vi "S2C_InitMenuItems.vi"(8 "Error In":errorcluster) -> (0 "Error Out":errorcluster)   [LabVIEW 2015]
doc: "Toggles the \"Local File\" runtime menu item."
uses:
  Globals/S2C_Globals.vi
  Globals/S2C_GlobalMenus.vi
  LVIS/Sub VIs/Globals/LVIS_DcGlobals.vi
  XML/S2C_XML_Globals.vi
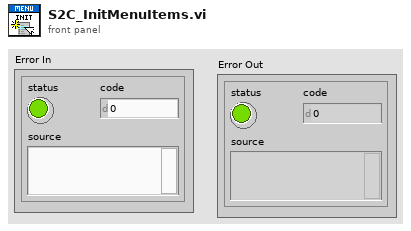
[diagram p1: front panel]
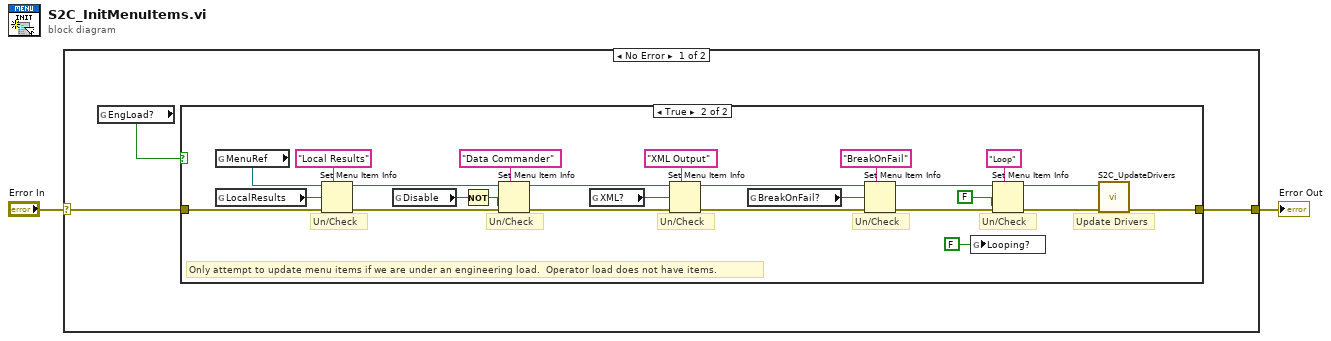
[diagram p0: block diagram]
diagram:
  n1 = case shown="No Error" "Error In" {
    selector: "Error In" -> [w5 w32]
    tunnel: [w4 w32] -> w1
    frame No Error {
      n2 = global read "S2C_Globals.vi" "EngLoad?"() -> (w3:bool)
      n3 = case shown="True" w3 {
        tunnel: w5 -> [w6 w24]
        tunnel: [w6 w23] -> w4
        frame False {
          # "Running under operator load"
        }
        frame True {
          # "Un/Check"
          # "Un/Check"
          # "Only attempt to update menu items if we are under an engineering load.  Operator load does not have items."
          # "Un/Check"
          # "Update Drivers"
          # "Un/Check"
          # "Un/Check"
          n4 = global read "S2C_GlobalMenus.vi" "MenuRef"() -> (w25:refnum<k9>)
          n5 = global read "S2C_Globals.vi" "LocalResults"() -> (w31:bool)
          n6 = Set Menu Item Info(6:w31, 7:"Local Results" ("item tag"), 8:w24, 11:w25) -> (0:w29:errorcluster, 3:w26:refnum<k9>)  [unwired: 3 in]
          n7 = global read "LVIS_DcGlobals.vi" "Disable"() -> (w28:bool)
          n8 = Not(x=w28) -> (.not. x?=w27:bool)
          n9 = Set Menu Item Info(6:w27, 7:"Data Commander" ("item tag"), 8:w29, 11:w26) -> (0:w16:errorcluster, 3:w17:refnum<k9>)  [unwired: 3 in]
          n10 = global read "S2C_XML_Globals.vi" "XML?"() -> (w14:bool)
          n11 = Set Menu Item Info(6:w14, 7:"XML Output" ("item tag"), 8:w16, 11:w17) -> (0:w11:errorcluster, 3:w10:refnum<k9>)  [unwired: 3 in]
          n12 = global read "S2C_Globals.vi" "BreakOnFail?"() -> (w13:bool)
          n13 = Set Menu Item Info(6:w13, 7:"BreakOnFail" ("item tag"), 8:w11, 11:w10) -> (0:w9:errorcluster, 3:w8:refnum<k9>)  [unwired: 3 in]
          n14 = global write "S2C_Globals.vi" "Looping?"(FALSE ("Looping?")) -> ()
          n15 = Set Menu Item Info(6:FALSE, 7:"Loop" ("item tag"), 8:w9, 11:w8) -> (0:w15:errorcluster, 3:w20:refnum<k9>)  [unwired: 3 in]
          n16 = call "S2C_UpdateDrivers.vi"("Error In"=w15, "MenuRef"=w20) -> ("Error Out"=w23:errorcluster)  [unwired: 9 in]
        }
      }
    }
    frame Error {
    }
  }
  "Error Out" <- w1
